vi "Open VI by ref.vi"(8 "error in (no error)":errorcluster, 10 "reference":refnum<vi>, 11 "LV RT in":refnum<class "LV RT.lvclass">) -> (0 "error out":errorcluster, 3 "LV RT out":refnum<class "LV RT.lvclass">)   [LabVIEW 2019, in "LV RT.lvclass"]
uses:
  LV RT.lvclass
  D:/Namratha/MDI/LabVIEW-MDI-develop_LV2019/source code/Document/LV Doc/LV Doc.lvclass
  LV Doc.lvclass/LV Doc.ctl
  LV RT.lvclass/LV RT.ctl
  property/Write VI Reference.vi
  property/Write Instantiated by ref_.vi
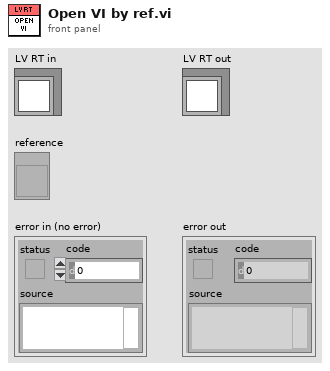
[diagram p1: front panel]
types:
  T1 = enum32{"Invalid", "Standard", "Closed", "Hidden", "Minimized", "Maximized"}
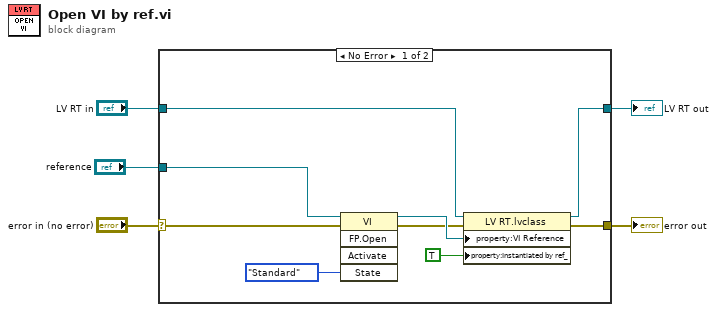
[diagram p0: block diagram]
diagram:
  n1 = case shown="No Error" "error in (no error)" {
    selector: "error in (no error)" -> [w8 w16]
    tunnel: [w9 w16] -> w4
    tunnel: [w11 w15] -> w2
    tunnel: "LV RT in" -> [w12 w15]
    tunnel: "reference" -> [w7 _]
    frame No Error {
      n2 = invoke class="VI" method="FP.Open"(reference=w7, error in=w8, "State"=T1."Standard") -> (reference out=w13:refnum<vi>, error out=w10:errorcluster)  [unwired: 2 in, 3 out]
      n3 = property class="LV RT.lvclass"(reference=w12, error in=w10, "property:VI Reference"=w13, "property:Instantiated by ref_"=TRUE ("Instantiated by ref_")) -> (reference out=w11:refnum<class "LV RT.lvclass">, error out=w9:errorcluster)
    }
    frame Error {
    }
  }
  "error out" <- w4
  "LV RT out" <- w2
